vi "Bus Interface.vi"(0 "WaveformAddressSpace":refnum<class "WaveformAddressSpace.lvclass">, 1 "abort":bool, 5 "instruction":T2, 9 "input valid":bool) -> (6 "response":T1, 10 "done":bool, 14 "ready for input":bool)   [LabVIEW 2015, in "WaveformAddressSpace.lvclass"]
uses:
  WaveformAddressSpace.lvclass
  <instrlib>/_niInstr/Instruction Framework/v1/FPGA/Interfaces/Address Space/Address Space Instruction.ctl
  <instrlib>/_niInstr/Instruction Framework/v1/FPGA/Typedefs/Response.ctl
  WaveformAddressSpace.lvclass/WaveformAddressSpace.ctl
  <vilib>/rvi/DataTransferAndStorage/Container/Common/niFpgaContainerExecOnDevCompGetState.vi
  <vilib>/rvi/Emulation/niFpgaEmulationIsFPGAContextNoSignature.vi
  <vilib>/rvi/DataTransferAndStorage/Container/Common/niFpgaContainerGetUniqueNameForEmu.vi
  <vilib>/rvi/Memory/Memory_Emulation/niFpgaMemoryEmulationCacheClearOnFirstRun.vi
  <vilib>/rvi/Memory/Memory_Emulation/nirvimemoryEmulationManagerCache_MakeExclusive.vi
  <vilib>/rvi/Memory/Memory_Emulation/niFpgaMemoryEmulationValidateCache.vi
  <vilib>/rvi/Memory/Memory_Emulation/nirvimemoryEmulationManagerCache_InsertValue.vi
  <vilib>/Utility/error.llb/Clear Errors.vi
  <vilib>/rvi/Memory/Memory_Emulation/nirvimemoryEmulationManagerCache_ReleaseExclusive.vi
  <vilib>/rvi/Memory/Memory_Emulation/nirvimemoryEmulationManagerCache_GetValue.vi
  <vilib>/rvi/Memory/Memory_Emulation/nirvimemoryEmulationManagerCache_SetValue.vi
  <vilib>/rvi/Emulation/niFpgaProcessEmulError.vi
  <vilib>/rvi/Emulation/niFpgaSctlEmulationGetInTimedLoop.vi
  <vilib>/rvi/DataTransferAndStorage/Container/XNode/niFpgaContainer.xnode
  <vilib>/rvi/DataTransferAndStorage/Register/Emulation/niFpgaRegisterEmulationRefIn.vi
  <instrlib>/_niInstr/Instruction Framework/v1/FPGA/Typedefs/niInstr Instruction Framework v1 FPGA.lvlib
  <instrlib>/_niInstr/Instruction Framework/v1/FPGA/Interfaces/Address Space/Address Space.lvclass
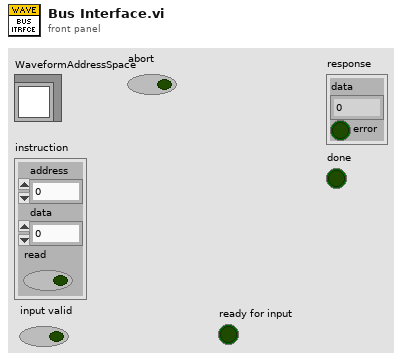
[diagram p1: front panel]
types:
  T1 = typedef "niInstr Instruction Framework v1 FPGA.lvlib/Response.ctl" = cluster{"data":u64, "error":bool}
  T2 = typedef "niInstr Instruction Framework Interfaces v1 FPGA.lvlib/Address Space.lvclass/Address Space Instruction.ctl" = cluster{"address":u32, "data":u64, "read":bool}
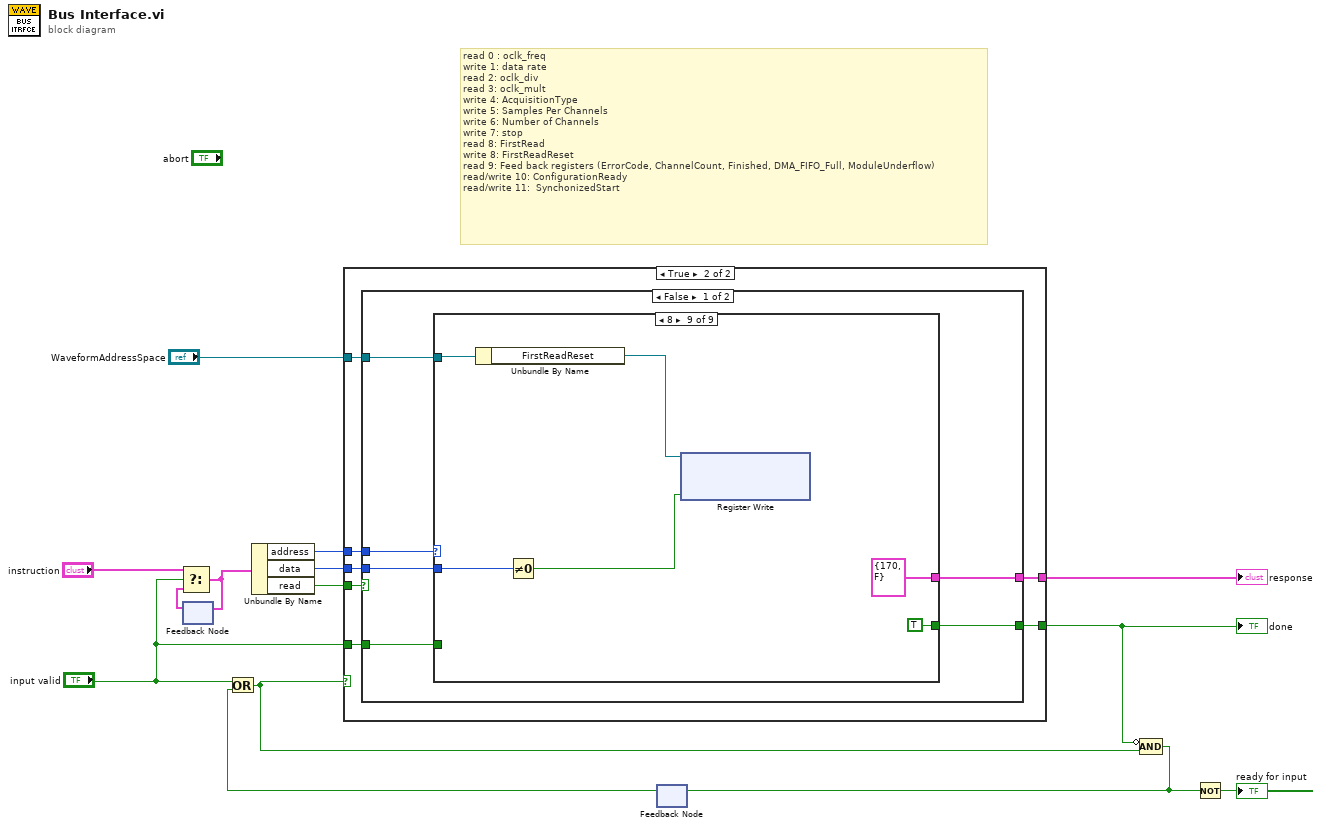
[diagram p0: block diagram]
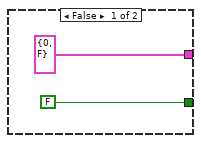
[diagram p2: hidden frame]
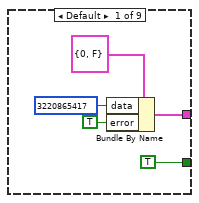
[diagram p3: hidden frame]
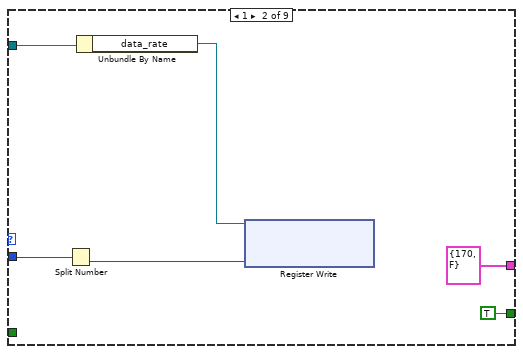
[diagram p4: hidden frame]
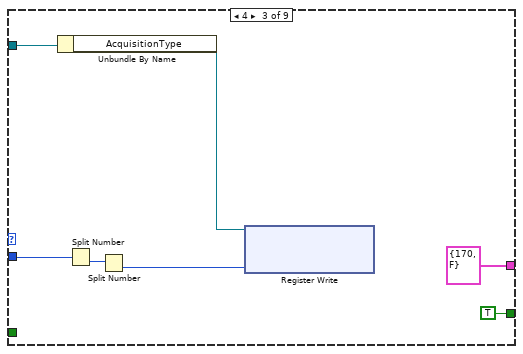
[diagram p5: hidden frame]
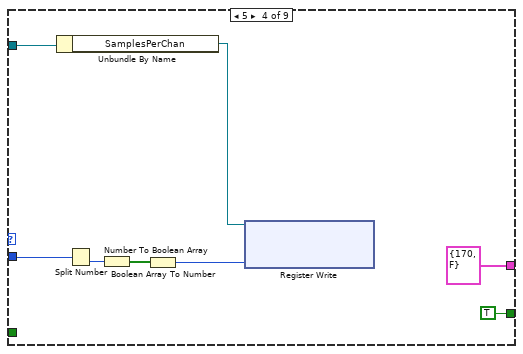
[diagram p6: hidden frame]
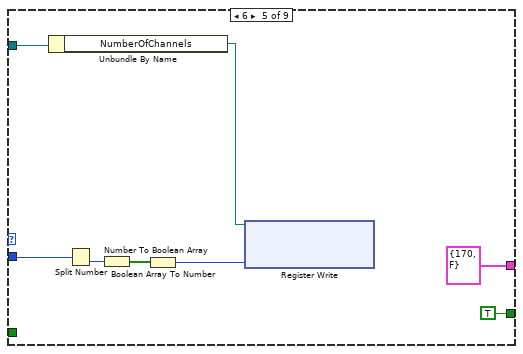
[diagram p7: hidden frame]
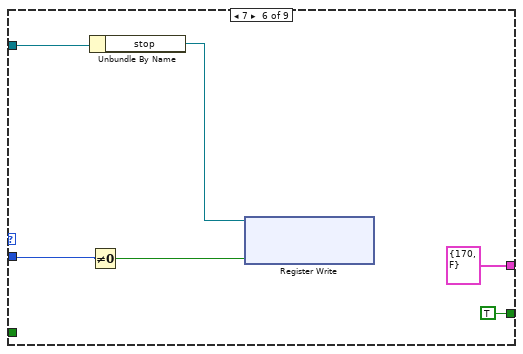
[diagram p8: hidden frame]
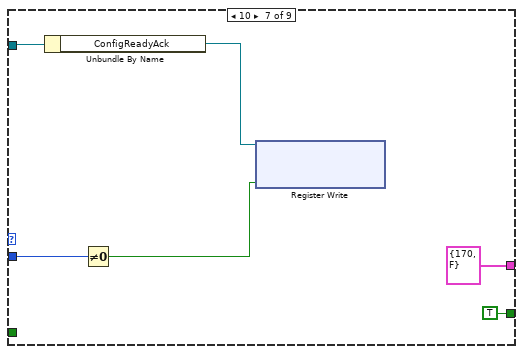
[diagram p9: hidden frame]
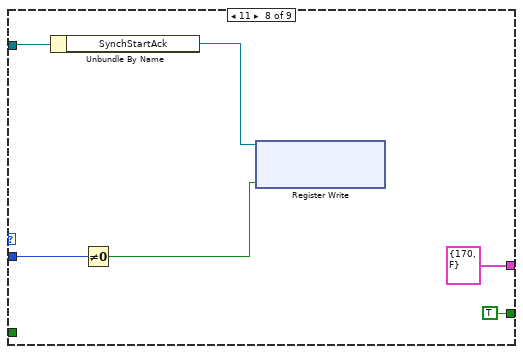
[diagram p10: hidden frame]
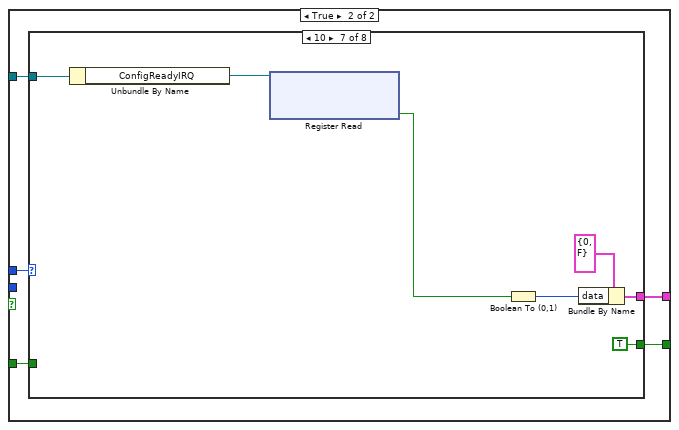
[diagram p11: hidden frame]
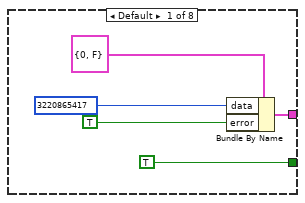
[diagram p12: hidden frame]
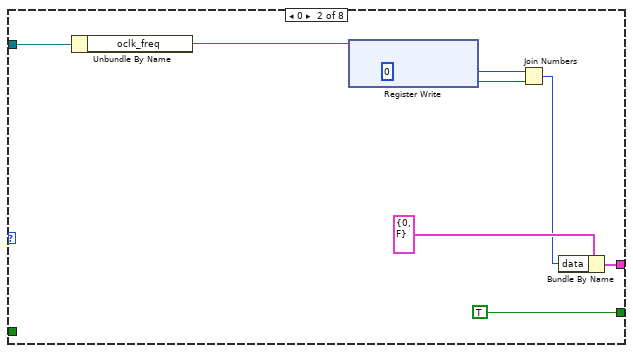
[diagram p13: hidden frame]
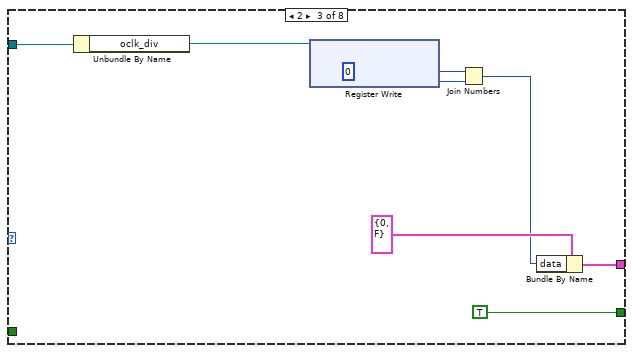
[diagram p14: hidden frame]
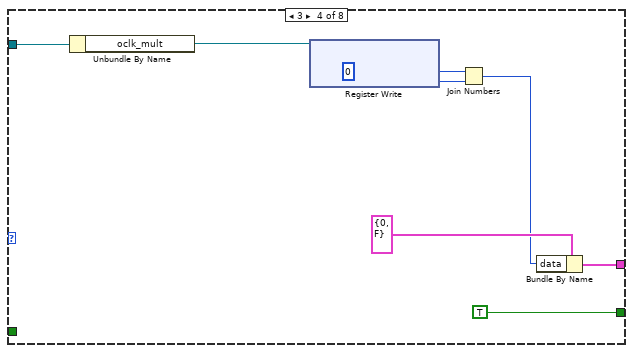
[diagram p15: hidden frame]
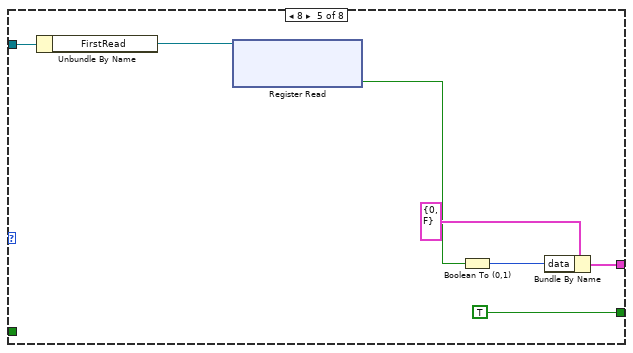
[diagram p16: hidden frame]
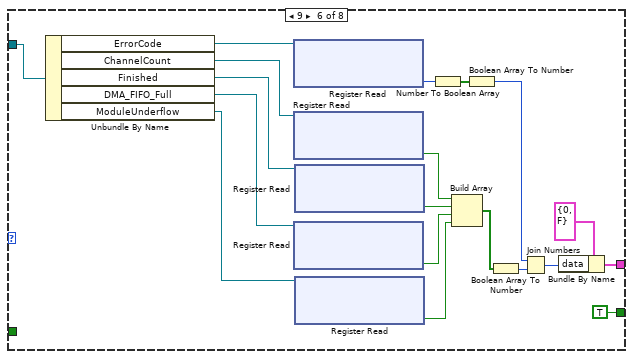
[diagram p17: hidden frame]
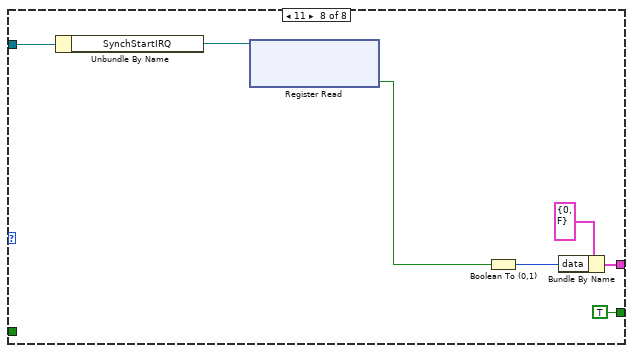
[diagram p18: hidden frame]
diagram:
  # "read 0 : oclk_freq\nwrite 1: data rate\nread 2: oclk_div\nread 3: oclk_mult\nwrite 4: AcquisitionType\nwrite 5: Samples Per Channels\nwrite 6: Number of Channels\nwrite 7: stop\nread 8: FirstRead\nwrite 8: FirstReadReset\nread 9: Feed back registers (ErrorCode, ChannelCount, Finished, DMA_FIFO_Full, ModuleUnderflow)\nread/write 10: ConfigurationReady\nread/write 11:  SynchonizedStart"
  n1 = feedback #1() -> (w14:T2)  [unwired: 1 in]
  n2 = Select(t="instruction", s="input valid", f=w14) -> (s? t:f=w13:T2)
  n3 = feedback-in #1(w13) -> ()
  n4 = Unbundle By Name(w13) -> ("address"=w10:u32, "data"=w11:u64, "read"=w12:bool)
  n5 = feedback #2() -> (w7:bool)  [unwired: 1 in]
  n6 = Or(x="input valid", y=w7) -> (x .or. y?=w8:bool)
  n7 = case shown="True" w8 {
    tunnel: w12 -> [_ w23]
    tunnel: w10 -> [_ w22]
    tunnel: w11 -> [_ w21]
    tunnel: [T1 {"data"=0, "error"=FALSE} ("response") w20] -> w3
    tunnel: [FALSE ("Output Valid") w19] -> w2
    tunnel: "WaveformAddressSpace" -> [_ w18]
    tunnel: "input valid" -> [_ w17]
    frame False {
    }
    frame True {
      n8 = case shown="False" w23 {
        tunnel: w22 -> [w29 w92]
        tunnel: w21 -> [w28 _]
        tunnel: [w27 w91] -> w20
        tunnel: [w26 w90] -> w19
        tunnel: w18 -> [w25 w89]
        tunnel: w17 -> [w24 w88]
        frame False {
          n9 = case shown="8" w29 {
            tunnel: w28 -> [_ w36 w43 w51 w59 w65 w71 w77 w83]
            tunnel: [w31 T1 {"data"=170, "error"=FALSE} ("response") T1 {"data"=170, "error"=FALSE} ("response") T1 {"data"=170, "error"=FALSE} ("response") T1 {"data"=170, "error"=FALSE} ("response") T1 {"data"=170, "error"=FALSE} ("response") T1 {"data"=170, "error"=FALSE} ("response") T1 {"data"=170, "error"=FALSE} ("response") T1 {"data"=170, "error"=FALSE} ("response")] -> w27
            tunnel: [TRUE ("done") TRUE ("done") TRUE ("done") TRUE ("done") TRUE ("done") TRUE ("done") TRUE ("done") TRUE ("done") TRUE ("done")] -> w26
            tunnel: w25 -> [_ w38 w45 w53 w61 w67 w75 w81 w87]
            tunnel: w24 -> [_ _ _ _ _ _ _ _ _]
            frame Default {
              n10 = Bundle By Name(cluster=T1 {"data"=0, "error"=FALSE} ("response"), "data"=u64 3220865417, "error"=TRUE) -> (w31:T1)
            }
            frame 1 {
              n11 = Split Number(x=w36) -> (lo(x)=w35:u32)  [unwired: 1 out]
              n12 = Unbundle By Name(w38) -> ("data_rate"=w37:refnum<k21>)
              n13 = xnode ("Register Write")("Data"=w35, "Register In"=w37) -> ()  [unwired: 1 out]
            }
            frame 4 {
              n14 = Unbundle By Name(w45) -> ("AcquisitionType"=w44:refnum<k21>)
              n15 = Split Number(x=w43) -> (lo(x)=w42:u32)  [unwired: 1 out]
              n16 = Split Number(x=w42) -> (lo(x)=w41:u16)  [unwired: 1 out]
              n17 = xnode ("Register Write")("Data"=w41, "Register In"=w44) -> ()  [unwired: 1 out]
            }
            frame 5 {
              n18 = Unbundle By Name(w53) -> ("SamplesPerChan"=w52:refnum<k21>)
              n19 = Split Number(x=w51) -> (lo(x)=w50:u32)  [unwired: 1 out]
              n20 = Number To Boolean Array(number=w50) -> (Boolean array=w49:bool[])
              n21 = Boolean Array To Number(Boolean array=w49) -> (number=w48:i32)
              n22 = xnode ("Register Write")("Data"=w48, "Register In"=w52) -> ()  [unwired: 1 out]
            }
            frame 6 {
              n23 = Unbundle By Name(w61) -> ("NumberOfChannels"=w60:refnum<k21>)
              n24 = Split Number(x=w59) -> (lo(x)=w58:u32)  [unwired: 1 out]
              n25 = Number To Boolean Array(number=w58) -> (Boolean array=w57:bool[])
              n26 = Boolean Array To Number(Boolean array=w57) -> (number=w56:i32)
              n27 = xnode ("Register Write")("Data"=w56, "Register In"=w60) -> ()  [unwired: 1 out]
            }
            frame 7 {
              n28 = Unbundle By Name(w67) -> ("stop"=w66:refnum<k21>)
              n29 = Not Equal To 0?(x=w65) -> (x != 0?=w64:bool)
              n30 = xnode ("Register Write")("Data"=w64, "Register In"=w66) -> ()  [unwired: 1 out]
            }
            frame 10 {
              n31 = Unbundle By Name(w75) -> ("ConfigReadyAck"=w72:refnum<k21>)
              n32 = Not Equal To 0?(x=w71) -> (x != 0?=w70:bool)
              n33 = xnode ("Register Write")("Data"=w70, "Register In"=w72) -> ()  [unwired: 1 out]
            }
            frame 11 {
              n34 = Unbundle By Name(w81) -> ("SynchStartAck"=w78:refnum<k21>)
              n35 = Not Equal To 0?(x=w77) -> (x != 0?=w76:bool)
              n36 = xnode ("Register Write")("Data"=w76, "Register In"=w78) -> ()  [unwired: 1 out]
            }
            frame 8 {
              n37 = Unbundle By Name(w87) -> ("FirstReadReset"=w84:refnum<k21>)
              n38 = Not Equal To 0?(x=w83) -> (x != 0?=w82:bool)
              n39 = xnode ("Register Write")("Data"=w82, "Register In"=w84) -> ()  [unwired: 1 out]
            }
          }
        }
        frame True {
          n40 = case shown="10" w92 {
            tunnel: [w94 w98 w106 w114 w124 w143 w151 w158] -> w91
            tunnel: [TRUE ("done") TRUE ("done") TRUE ("done") TRUE ("done") TRUE ("done") TRUE ("done") TRUE ("done") TRUE ("done")] -> w90
            tunnel: w89 -> [_ w104 w112 w120 w128 w147 w154 w161]
            tunnel: w88 -> [_ _ _ _ _ _ _ _]
            frame Default {
              n41 = Bundle By Name(cluster=T1 {"data"=0, "error"=FALSE} ("response"), "data"=u64 3220865417, "error"=TRUE) -> (w94:T1)
            }
            frame 0 {
              n42 = Unbundle By Name(w104) -> ("oclk_freq"=w105:refnum<k21>)
              n43 = xnode ("Register Write")("Register In"=w105) -> ("Data"=w103:u32)  [unwired: 1 out]
              n44 = Join Numbers(hi=u32 0, lo=w103) -> ((hi.lo)=w99:u64)
              n45 = Bundle By Name(cluster=T1 {"data"=0, "error"=FALSE} ("response"), "data"=w99) -> (w98:T1)
            }
            frame 2 {
              n46 = Unbundle By Name(w112) -> ("oclk_div"=w113:refnum<k21>)
              n47 = xnode ("Register Write")("Register In"=w113) -> ("Data"=w111:u32)  [unwired: 1 out]
              n48 = Join Numbers(hi=u32 0, lo=w111) -> ((hi.lo)=w107:u64)
              n49 = Bundle By Name(cluster=T1 {"data"=0, "error"=FALSE} ("response"), "data"=w107) -> (w106:T1)
            }
            frame 3 {
              n50 = Unbundle By Name(w120) -> ("oclk_mult"=w121:refnum<k21>)
              n51 = xnode ("Register Write")("Register In"=w121) -> ("Data"=w119:u32)  [unwired: 1 out]
              n52 = Join Numbers(hi=u32 0, lo=w119) -> ((hi.lo)=w115:u64)
              n53 = Bundle By Name(cluster=T1 {"data"=0, "error"=FALSE} ("response"), "data"=w115) -> (w114:T1)
            }
            frame 8 {
              n54 = Unbundle By Name(w128) -> ("FirstRead"=w127:refnum<k21>)
              n55 = xnode ("Register Read")("Register In"=w127) -> ("Data"=w123:bool)  [unwired: 1 out]
              n56 = Boolean To (0,1)(Boolean=w123) -> (0, 1=w122:i16)
              n57 = Bundle By Name(cluster=T1 {"data"=0, "error"=FALSE} ("response"), "data"=w122) -> (w124:T1)
            }
            frame 9 {
              n58 = Unbundle By Name(w147) -> ("ErrorCode"=w146:refnum<k21>, "ChannelCount"=w138:refnum<k21>, "Finished"=w137:refnum<k21>, "DMA_FIFO_Full"=w136:refnum<k21>, "ModuleUnderflow"=w135:refnum<k21>)
              n59 = xnode ("Register Read")("Register In"=w146) -> ("Data"=w142:i32)  [unwired: 1 out]
              n60 = xnode ("Register Read")("Register In"=w138) -> ("Data"=w134:bool)  [unwired: 1 out]
              n61 = xnode ("Register Read")("Register In"=w136) -> ("Data"=w132:bool)  [unwired: 1 out]
              n62 = xnode ("Register Read")("Register In"=w137) -> ("Data"=w133:bool)  [unwired: 1 out]
              n63 = xnode ("Register Read")("Register In"=w135) -> ("Data"=w131:bool)  [unwired: 1 out]
              n64 = Number To Boolean Array(number=w142) -> (Boolean array=w141:bool[])
              n65 = Build Array(w134, w133, w132, w131) -> (w130:bool[])
              n66 = Boolean Array To Number(Boolean array=w141) -> (number=w139:u32)
              n67 = Boolean Array To Number(Boolean array=w130) -> (number=w129:u32)
              n68 = Join Numbers(hi=w139, lo=w129) -> ((hi.lo)=w140:u64)
              n69 = Bundle By Name(cluster=T1 {"data"=0, "error"=FALSE} ("response"), "data"=w140) -> (w143:T1)
            }
            frame 10 {
              n70 = Unbundle By Name(w154) -> ("ConfigReadyIRQ"=w150:refnum<k21>)
              n71 = xnode ("Register Read")("Register In"=w150) -> ("Data"=w149:bool)  [unwired: 1 out]
              n72 = Boolean To (0,1)(Boolean=w149) -> (0, 1=w148:i16)
              n73 = Bundle By Name(cluster=T1 {"data"=0, "error"=FALSE} ("response"), "data"=w148) -> (w151:T1)
            }
            frame 11 {
              n74 = Unbundle By Name(w161) -> ("SynchStartIRQ"=w157:refnum<k21>)
              n75 = xnode ("Register Read")("Register In"=w157) -> ("Data"=w156:bool)  [unwired: 1 out]
              n76 = Boolean To (0,1)(Boolean=w156) -> (0, 1=w155:i16)
              n77 = Bundle By Name(cluster=T1 {"data"=0, "error"=FALSE} ("response"), "data"=w155) -> (w158:T1)
            }
          }
        }
      }
    }
  }
  "done" <- w2
  "response" <- w3
  n78 = Compound Arithmetic op=AND(invert w2, w8) -> (w9:bool)
  n79 = feedback-in #2(w9) -> ()
  n80 = Not(x=w9) -> (.not. x?=→"ready for input":bool)
